vi "Python_Logic2_Automation-Analog.vi"() -> ()   [LabVIEW 2021]
doc: "This example demonstrates how to use Python to control the Ssaleae Logic2 software supporting the Logic 8, Logic Pro 8 and Logic Pro 16 logic annalyzers."
uses:
  <vilib>/Utility/sysdir.llb/System Directory Type.ctl
  <vilib>/Python/Open Anaconda Python Session.vi
  <vilib>/Utility/file.llb/Read Delimited Spreadsheet (DBL).vi
panel:
  out "XY Graph":cluster{"all rows":dbl[], "all rows":dbl[]}(graph)
  in  "Analog Config":T1={"Enable Analog Channels"=[0], "Analog Sample Rate (Samp/Sec)"=3125000} {"Analog Sample Rate (Samp/Sec)" format="%#.4p"}
  in  "Save Data?":bool=TRUE
  out "Saleae Capture":string
  out "Raw Analog":string
  in  "Device ID":string="F4241"
  in  "Capture Duration (s)":dbl=0.1 format="%^#_13g"
  in  "Port [10430]":i32=10430
  in  "IP Address [127.0.0.1]":string="127.0.0.1"
  out "Anaconda3 Path":path
  in  "Python version":string="3.8"
  in  "Anaconda Environment":string="Python38"
  out "error out":errorcluster
  in  "error in (no error)":errorcluster
  # "1. Python Settings"
  # "2. Logic2 Automation Server"
  # "3. Configure Device"
  # "4. Configure Capture"
  # "5. Start Capture"
  # "6. Add SPI Analyzer"
  # "7. Saved Files"
  # "Overview: Demonstrates how to use Python to automate the Saleae Logic2 software.\nRequirements: Python 3.8, 3.9 or 3.10 with the same bitness as LabVIEW.\nInstructions:\n1. Install LabVIEW, and setup an Anaconda 3 instance using Python 3.8\n  https://knowledge.ni.com/KnowledgeArticleDetails?id=kA00Z0000015C6tSAE&l=en-US \n2. Install the Saleae Python library using the instructions found here:\n  https://saleae.github.io/logic2-automation/getting_started.html#installing-the-python-automation-api-package\n# 3. Be sure Automation is enabled in the Logic2 Software (Saleae link above)\n# 4. The key parameters in this VI are the Anaconda setup and the Saleae 'Device ID' (F4241 is the default simulated Logic Pro 16)"
  # "Options: 50M, 12.5M, 6.25M, 3.125M, 1.5625M, 781.25k, 31.25k, 15.625k, 6.25k, 3.125M\n(Analog and Digital Rates must be multiples)"
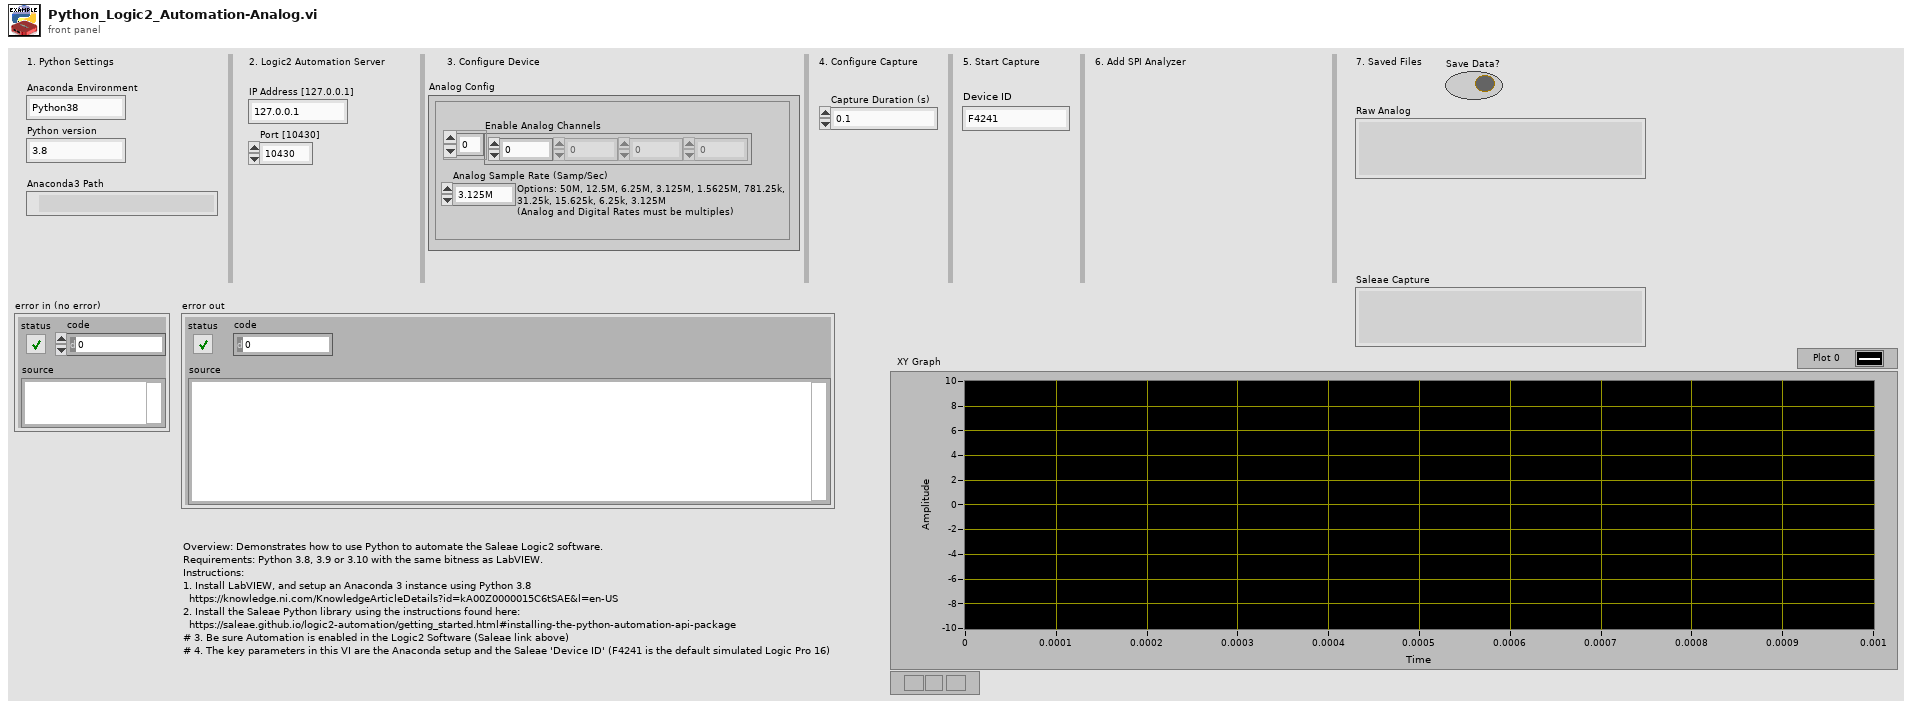
[diagram p1: front panel]
types:
  T1 = cluster{"Enable Analog Channels":i32[], "Analog Sample Rate (Samp/Sec)":i32}
  T2 = typedef "System Directory Type.ctl" = i32
  T3 = cluster{"Refnum in":refnum<k35>, "Python Module Name":path}
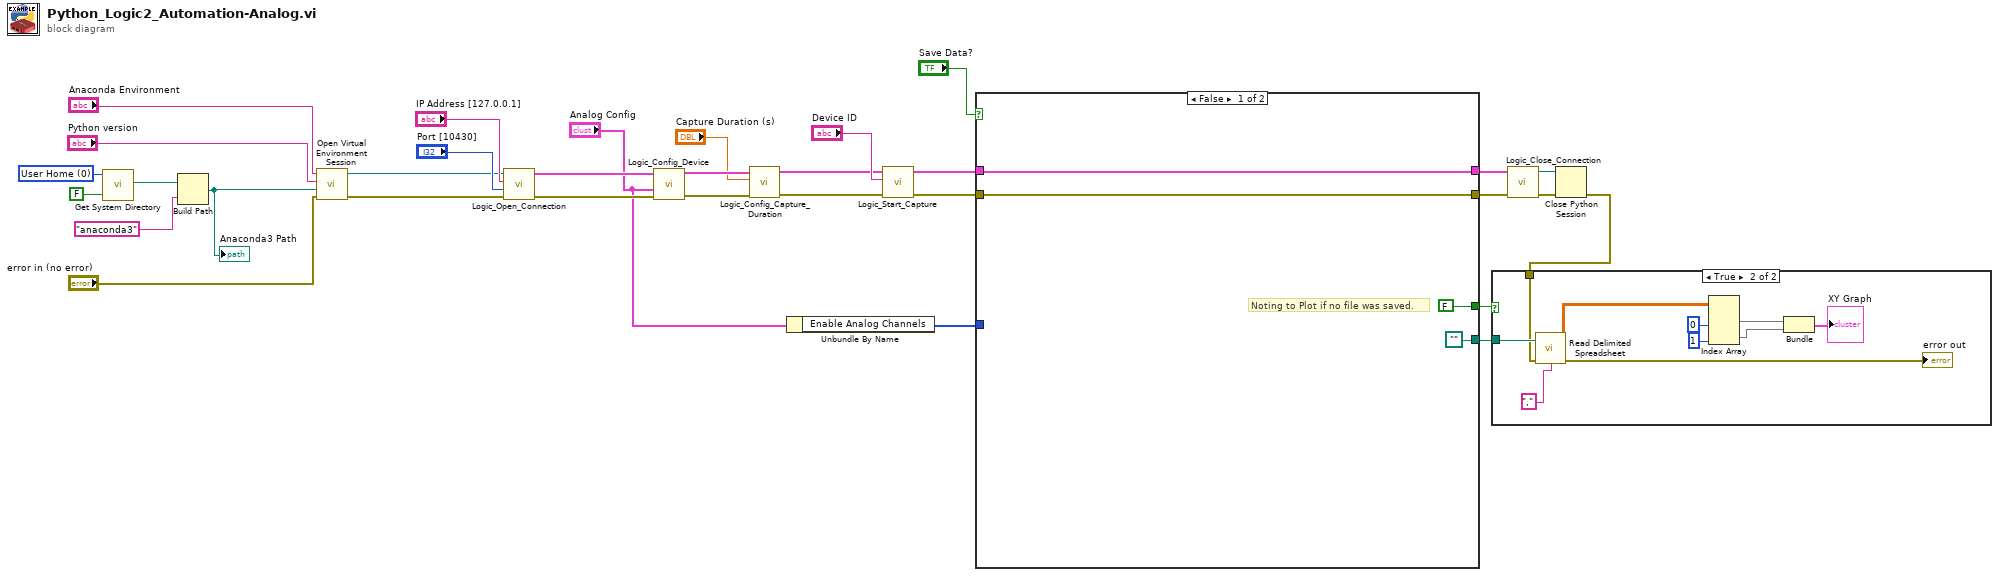
[diagram p0: block diagram]
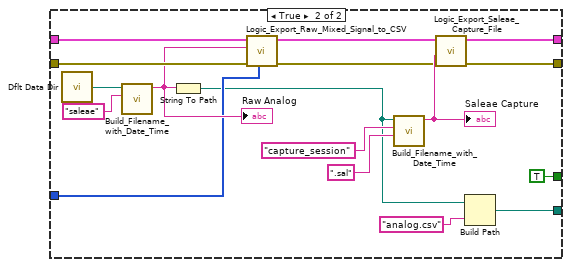
[diagram p3: hidden frame]
diagram:
  w27 = T2 0 items=["User Home"=0, "User Desktop"=1, "User Documents"=2, "User Application Data"=3, "User Preferences"=4, "User Temporary"=5, "Public Documents"=6, "Public Application Data"=7, "Public Preferences"=8, "Public Cache"=13, "System Core Libraries"=9, "System Installed Libraries"=10, "Application Files"=11, "Boot Volume Root"=12] ("system directory type")
  n1 = call <vilib>:"Get System Directory.vi"("create directory if not found? (F)"=FALSE, "system directory type"=w27) -> ("system directory"=w25:path)  [unwired: 9 in]
  n2 = Build Path(base path=w25, name or relative path="anaconda3") -> (appended path=w28:path)
  "Anaconda3 Path" <- w28
  n3 = call-poly <vilib>:"Open Virtual Environment Session.vi"("error in (no error)"="error in (no error)", "Anaconda path"=w28, "Python version"="Python version", "Env name"="Anaconda Environment") -> ("error out"=w15:errorcluster, "session out"=w16:refnum<k35>)  [unwired: 6 in]
  n4 = call "Logic_Open_Connection.vi"("error in (no error)"=w15, "Port [10430]"="Port [10430]", "IP Address [127.0.0.1]"="IP Address [127.0.0.1]", "Python Session In"=w16) -> ("error out"=w13:errorcluster, "Session Ref Out"=w19:T3)  [unwired: 2 in]
  n5 = call "Logic_Config_Device.vi"("error in (no error)"=w13, "Analog Config"="Analog Config", "Session Ref In"=w19) -> ("error out"=w20:errorcluster, "Session Ref Out"=w22:T3)  [unwired: 3 in]
  n6 = call "Logic_Config_Capture_Duration.vi"("error in (no error)"=w20, "Capture Duration (s)"="Capture Duration (s)", "Session Ref In"=w22) -> ("error out"=w21:errorcluster, "Session Ref Out"=w23:T3)  [unwired: 3 in]
  n7 = Unbundle By Name("Analog Config") -> ("Enable Analog Channels"=w10:i32[])
  n8 = call "Logic_Start_Capture.vi"("error in (no error)"=w21, "Device ID"="Device ID", "Session Ref In"=w23) -> ("error out"=w4:errorcluster, "Session Ref Out"=w5:T3)  [unwired: 3 in]
  n9 = case shown="False" "Save Data?" {
    tunnel: w4 -> [w35 w53]
    tunnel: w5 -> [w36 w52]
    tunnel: w10 -> [_ w43]
    tunnel: [w36 w49] -> w9
    tunnel: [w35 w48] -> w8
    tunnel: [path "" ("appended path") w38] -> w3
    tunnel: [FALSE TRUE] -> w1
    frame False {
      # "Noting to Plot if no file was saved."
    }
    frame True {
      n10 = call <vilib>:"Dflt Data Dir.vi"() -> ("App:Default Data Directory"=w46:path)
      n11 = call "Build_Filename_with_Date_Time.vi"("Item Prefix"="saleae" ("Filename Prefx"), "Folder for Data Captures"=w46) -> ("File Path Output"=w44:string)  [unwired: 9 in]
      "Raw Analog" <- w44
      n12 = String To Path(string=w44) -> (path=w41:path)
      n13 = call "Logic_Export_Raw_Mixed_Signal_to_CSV.vi"("Enabled Analog Channels"=w43, "error in (no error)"=w53, "Filepath Input"=w44, "Session Ref In"=w52) -> ("error out"=w39:errorcluster, "Session Ref Out"=w42:T3)  [unwired: 6 in]
      n14 = call "Build_Filename_with_Date_Time.vi"("File Extension (.csv)"=".sal", "Item Prefix"="capture_session" ("Filename Prefx"), "Folder for Data Captures"=w41) -> ("File Path Output"=w47:string)  [unwired: 8 in]
      "Saleae Capture" <- w47
      n15 = call "Logic_Export_Saleae_Capture_File.vi"("error in (no error)"=w39, "Filepath Input"=w47, "Session Ref In"=w42) -> ("error out"=w48:errorcluster, "Session Ref Out"=w49:T3)  [unwired: 3 in]
      n16 = Build Path(base path=w41, name or relative path="analog.csv" ("Filename Prefx")) -> (appended path=w38:path)
    }
  }
  n17 = call "Logic_Close_Connection.vi"("error in (no error)"=w8, "Session Ref In"=w9) -> ("error out"=w11:errorcluster, "Python Session Out"=w12:refnum<k35>)  [unwired: 4 in]
  n18 = Close Python Session(session in=w12, error in=w11) -> (11:w2:errorcluster)
  n19 = case shown="True" w1 {
    tunnel: w3 -> [_ w58]
    tunnel: w2 -> [_ w55]
    frame False {
      # "Noting to Plot if no file was saved."
    }
    frame True {
      n20 = call-poly <vilib>:"Read Delimited Spreadsheet.vi"("file path (dialog if empty)"=w58, "error in (no error)"=w55, "delimiter (\\t)"="," ("delimiter (\\t)")) -> ("all rows"=w56:dbl[][], "error out"=→"error out":errorcluster)  [unwired: 7 in, 4 out]
      n21 = Index Array(array=w56, index (col) #1=0 ("disabled index (col)"), index (col) #2=1 ("index (col)")) -> (element #1=w61:dbl[], element #2=w60:dbl[])  [unwired: 2 in]
      n22 = Bundle("all rows"=w61, "all rows"=w60) -> (→"XY Graph":cluster{"all rows":dbl[], "all rows":dbl[]})  [unwired: 1 in]
    }
  }
